vi "ma_FRF Function no State.vi"(0 "time signal X":waveform(dbl), 1 "time signal Y":waveform(dbl), 2 "window parameter":dbl=nan, 3 "window":T3=1 items=["Rectangle"=0, "Hanning"=1, "Hamming"=2, "Blackman-Harris"=3, "Exact Blackman"=4, "Blackman"=5, "Flat Top"=6, "4 Term B-Harris "=7, "7 Term B-Harris"=8, "Low Sidelobe"=9, "Blackman Nuttall"=11, "Triangle"=30, "Bartlett-Hanning"=31, "Bohman"=32, "Parzen"=33, "Welch"=34, "Kaiser"=60, "Dolph-Chebyshev"=61, "Gaussian"=62], 4 "view":T1, 5 "error in (no error)":errorcluster, 6 "restart averaging (F)":bool, 7 "averaging parameters":T5={"averaging mode"=enum."No averaging", "weighting mode"=enum."Exponential", "number of averages"=10} {"number of averages" min=1}, 8 "mag-phase":bool, 9 "state info":T2 {"Syy" format="%0.2f"; "Sxy" format="%0.2f"; "Sy" format="%0.2f"; "Sxx" format="%0.2f"; "avgs completed" format="%0.2f"; "df" format="%0.2f"; "Sx" format="%0.2f"; "spectrum parameters"."window" items=["Rectangle"=0, "Hanning"=1, "Hamming"=2, "Blackman-Harris"=3, "Exact Blackman"=4, "Blackman"=5, "Flat Top"=6, "4 Term B-Harris "=7, "7 Term B-Harris"=8, "Low Sidelobe"=9, "Blackman Nuttall"=11, "Triangle"=30, "Bartlett-Hanning"=31, "Bohman"=32, "Parzen"=33, "Welch"=34, "Kaiser"=60, "Dolph-Chebyshev"=61, "Gaussian"=62]; "dt" format="%0.2f"; "timestamp" format="%0.2f"; "dt history" format="%0.2f"; "t0 history" format="%0.2f"}, 11 "FRF Mode":enum16{"H1", "H2", "H3"}(ring)) -> (12 "averaging done":bool, 13 "state info out":T2 {"Syy" format="%0.2f"; "Sxy" format="%0.2f"; "Sy" format="%0.2f"; "Sxx" format="%0.2f"; "avgs completed" format="%0.2f"; "df" format="%0.2f"; "Sx" format="%0.2f"; "spectrum parameters"."window" items=["Rectangle"=0, "Hanning"=1, "Hamming"=2, "Blackman-Harris"=3, "Exact Blackman"=4, "Blackman"=5, "Flat Top"=6, "4 Term B-Harris "=7, "7 Term B-Harris"=8, "Low Sidelobe"=9, "Blackman Nuttall"=11, "Triangle"=30, "Bartlett-Hanning"=31, "Bohman"=32, "Parzen"=33, "Welch"=34, "Kaiser"=60, "Dolph-Chebyshev"=61, "Gaussian"=62]; "dt" format="%0.2f"; "timestamp" format="%0.2f"; "dt history" format="%0.2f"; "t0 history" format="%0.2f"}, 14 "real or mag":cluster{"f0":dbl, "df":dbl, "real or mag":dbl[]} {"real or mag" format="%.2p"; "f0" format="%0.2p"; "df" format="%0.2p"}, 15 "imag or phase":T4 {"imag or phase" format="%.2p"; "f0" format="%0.2p"; "df" format="%0.2p"}, 17 "coherence":cluster{"f0":dbl, "df":dbl, "coherence":dbl[]}, 18 "averages completed":dbl format="%.2p", 19 "error out":errorcluster)   [LabVIEW 2020, in "NI_MAPro.lvlib"]
doc: "Computes the frequency response and the coherence based on the input signals. Results are returned as <B>real part</B>, <B>imaginary part</B>, and <B>coherence</B>."
uses:
  NI_MAPro.lvlib
  windowTd.ctl
  2-chan State.ctl
  NI_AALPro.lvlib
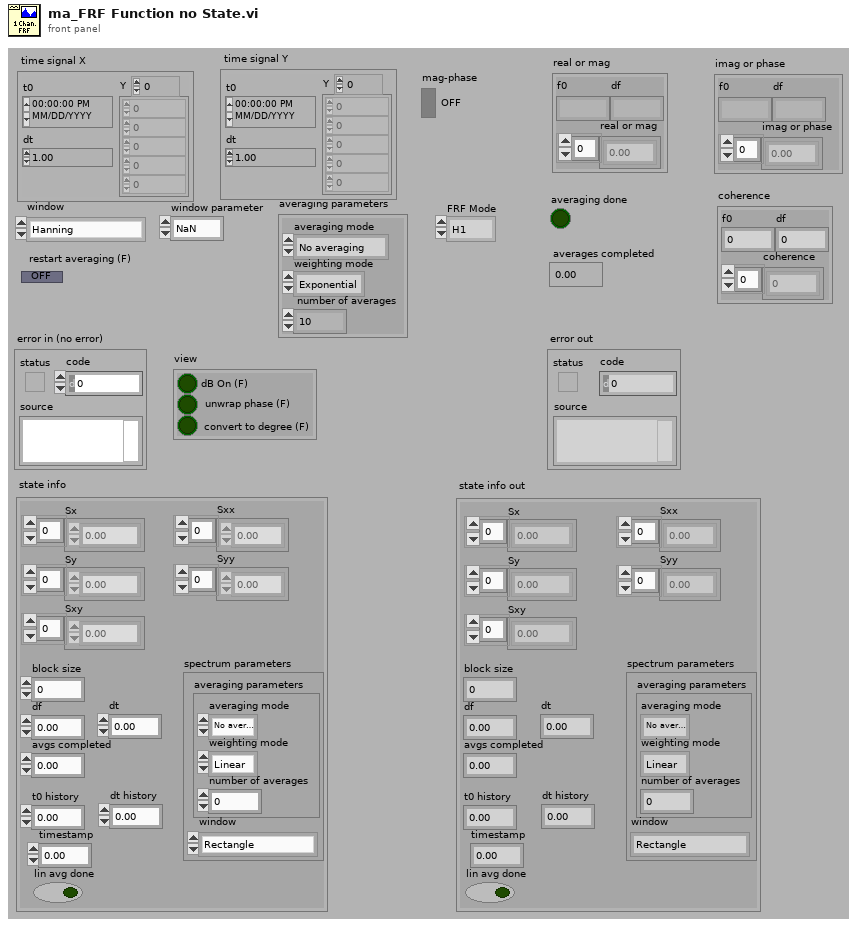
[diagram p1: front panel]
types:
  T1 = cluster{"dB On (F)":bool, "unwrap phase (F)":bool, "convert to degree (F)":bool}
  T2 = typedef "NI_MAPro.lvlib/2-chan State.ctl" = cluster{"Sx":cdb[], "Sy":cdb[], "Sxx":dbl[], "Syy":dbl[], "Sxy":cdb[], "block size":i32, "df":dbl, "dt":dbl, "avgs completed":dbl, "spectrum parameters":cluster{"averaging parameters":cluster{"averaging mode":enum16{"No averaging", "Vector averaging", "RMS averaging", "Peak hold"}, "weighting mode":enum16{"Linear", "Exponential"}, "number of averages":u32}, "window":T3}, "lin avg done":bool, "t0 history":dbl, "dt history":dbl, "timestamp":dbl}
  T3 = typedef "NI_AALPro.lvlib/windowTd.ctl" = u32
  T4 = cluster{"f0":dbl, "df":dbl, "imag or phase":dbl[]}
  T5 = cluster{"averaging mode":enum16{"No averaging", "Vector averaging", "RMS averaging", "Peak hold"}, "weighting mode":enum16{"Linear", "Exponential"}, "number of averages":u32}
  T6 = enum16{"FFT spectrum", "Power spectrum", "Cross spectrum", "Frequency response"}
  T7 = enum16{"No averaging", "Vector averaging", "RMS averaging", "Peak hold"}
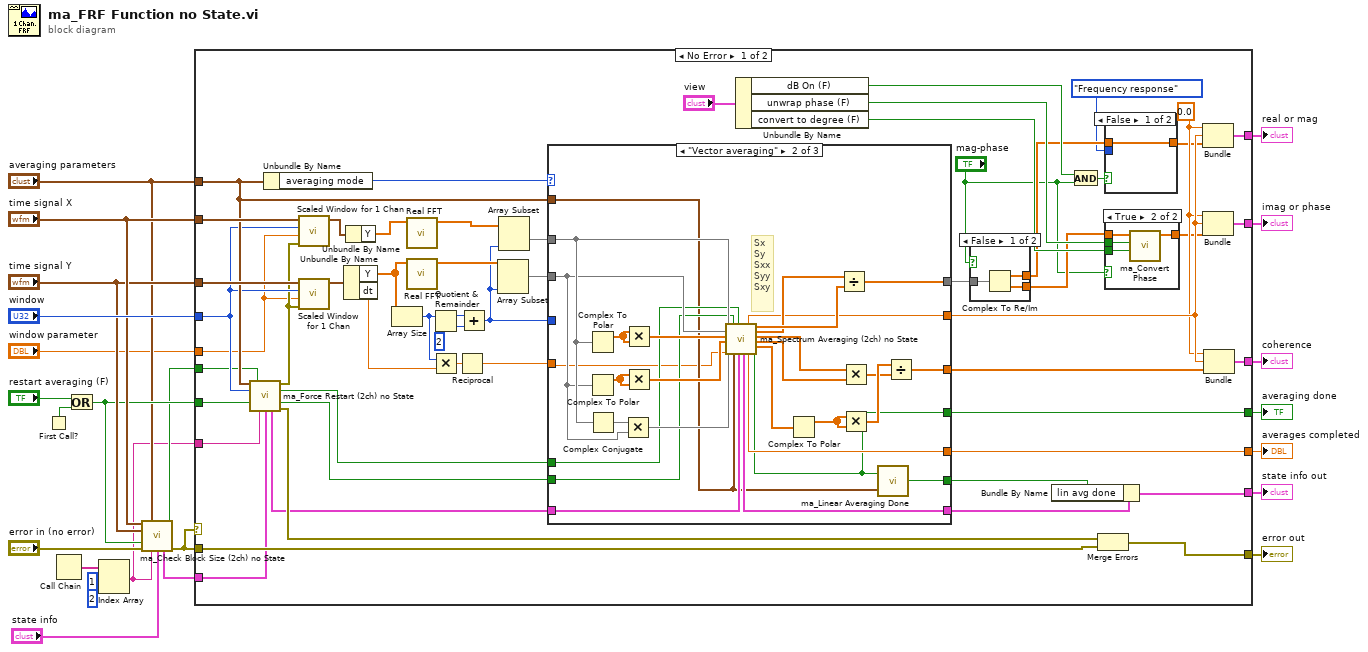
[diagram p0: block diagram]
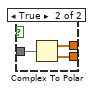
[diagram p2: hidden frame]
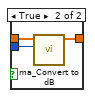
[diagram p4: hidden frame]
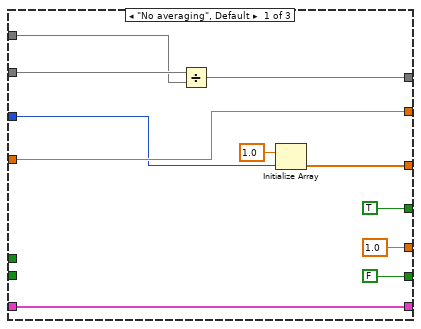
[diagram p5: hidden frame]
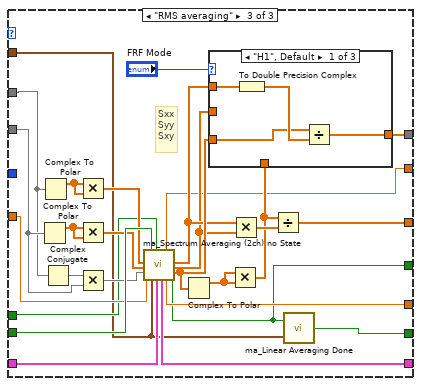
[diagram p6: hidden frame]
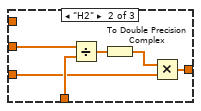
[diagram p7: hidden frame]
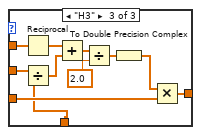
[diagram p8: hidden frame]
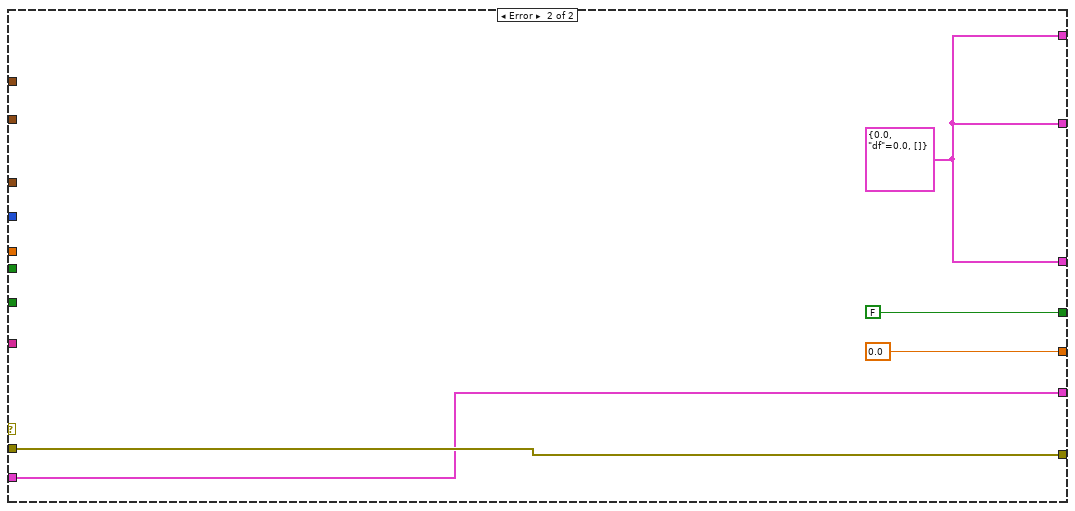
[diagram p9: hidden frame]
diagram:
  n1 = First Call?() -> (First Call?: T/F=w21:bool)
  n2 = Call Chain() -> (call chain=w6:string[])
  n3 = Or(x="restart averaging (F)", y=w21) -> (x .or. y?=w17:bool)
  n4 = Index Array(array=w6, index #1=1 ("Index"), index #2=2 ("Index")) -> (element #1=w5:string)  [unwired: 1 out]
  n5 = call "ma_Check Block Size (2ch) no State.vi"("time signal X"="time signal X", "averaging parameters"="averaging parameters", "time signal Y"="time signal Y", "restart averaging (F)"=w17, "error in"="error in (no error)", "caller VI name"=w5, "state info"="state info") -> ("force restart averaging"=w9:bool, "state info out"=w3:T2, "error out"=w14:errorcluster)  [unwired: 6 out]
  n6 = case shown="No Error" w14 {
    tunnel: [w80 0.0 ("averages completed")] -> w24
    tunnel: "time signal X" -> [w79 _]
    tunnel: "time signal Y" -> [w78 _]
    tunnel: [w77 FALSE ("averaging done")] -> w23
    tunnel: "averaging parameters" -> [w76 _]
    tunnel: "window" -> [w75 _]
    tunnel: w17 -> [w74 _]
    tunnel: [w67 w187] -> w15
    tunnel: w14 -> [w65 w187]
    tunnel: [w73 w185] -> w12
    tunnel: [w72 w185] -> w11
    tunnel: [w68 w185] -> w10
    tunnel: w5 -> [w64 _]
    tunnel: w9 -> [w63 _]
    tunnel: w3 -> [w62 w183]
    tunnel: [w39 w183] -> w2
    tunnel: "window parameter" -> [w25 _]
    frame No Error {
      w69 = 0.0
      n7 = call "ma_Force Restart (2ch) no State.vi"("averaging parameters"=w76, "force restart averaging in"=w63, "window"=w75, "restart averaging (F)"=w74, "caller VI name"=w64, "state info"=w62) -> ("skip processing"=w59:errorcluster, "force restart averaging"=w57:bool, "retrieve last spectrum"=w56:bool, "state info out"=w41:T2, "error out"=w66:errorcluster)  [unwired: 1 in, 4 out]
      n8 = Unbundle By Name(w76) -> ("averaging mode"=w58:T7)
      n9 = call "Scaled Window for 1 Chan.vi"("error in (no error)"=w59, "window parameter"=w25, "window"=w75, "signal in"=w79) -> ("signal out"=w60:waveform(dbl))  [unwired: 5 in, 2 out]
      n10 = call "Scaled Window for 1 Chan.vi"("error in (no error)"=w59, "window parameter"=w25, "window"=w75, "signal in"=w78) -> ("signal out"=w61:waveform(dbl))  [unwired: 5 in, 2 out]
      n11 = Unbundle By Name(w61) -> ("Y"=w46:dbl[], "dt"=w47:dbl)
      n12 = Unbundle By Name(w60) -> ("Y"=w45:dbl[])
      n13 = Array Size(array=w46) -> (size(s)=w55:i32)
      n14 = call "Real FFT.vi"("X"=w45) -> ("FFT {X}"=w53:cdb[])  [unwired: 9 in, 1 out]
      n15 = call "Real FFT.vi"("X"=w46) -> ("FFT {X}"=w54:cdb[])  [unwired: 9 in, 1 out]
      n16 = Quotient & Remainder(x=w55, y=2) -> (x-y*floor(x/y)=w50:i32, floor(x/y)=w49:i32)
      n17 = Multiply(x=w55, y=w47) -> (x*y=w52:dbl)
      n18 = Reciprocal(x=w52) -> (1/x=w48:dbl)
      n19 = Add(x=w50, y=w49) -> (x+y=w42:i32)
      n20 = Array Subset(array=w54, length=w42) -> (w43:cdb[])  [unwired: 1 in]
      n21 = Array Subset(array=w53, length=w42) -> (w44:cdb[])  [unwired: 1 in]
      n22 = case shown="\"Vector averaging\"" w58 {
        tunnel: [w100 w114 w137] -> w70
        tunnel: w57 -> [_ w115 w142]
        tunnel: w76 -> [_ w108 w135]
        tunnel: [1.0 ("averages completed") w116 w147] -> w80
        tunnel: [w105 w129 w160] -> w71
        tunnel: [TRUE ("averaging done") w113 w138] -> w77
        tunnel: w56 -> [_ w109 w148]
        tunnel: [FALSE ("linear averaging done") w131 w159] -> w40
        tunnel: w44 -> [w99 w126 w154]
        tunnel: w43 -> [w101 w125 w155]
        tunnel: w48 -> [w100 w107 w143]
        tunnel: w42 -> [w98 _ _]
        tunnel: w41 -> [w97 w112 w150]
        tunnel: [w97 w111 w149] -> w38
        tunnel: [w96 w110 w136] -> w30
        frame "No averaging", Default {
          n23 = Divide(x=w101, y=w99) -> (x/y=w96:cdb[])
          n24 = Initialize Array(1.0, w98) -> (w105:dbl[])
        }
        frame "Vector averaging" {
          # "Sx\nSy\nSxx\nSyy\nSxy"
          n25 = Complex To Polar(r * e^(i*theta)=w126) -> (r=w128:dbl[])  [unwired: 1 out]
          n26 = Complex To Polar(r * e^(i*theta)=w125) -> (r=w127:dbl[])  [unwired: 1 out]
          n27 = Complex Conjugate(1:w126) -> (0:w130:cdb[])
          n28 = Multiply(x=w130, y=w125) -> (x*y=w122:cdb[])
          n29 = Multiply(x=w128, y=w128) -> (x*y=w124:dbl[])
          n30 = Multiply(x=w127, y=w127) -> (x*y=w123:dbl[])
          n31 = call "ma_Spectrum Averaging (2ch) no State.vi"("Sx"=w126, "Sy"=w125, "Sxx"=w124, "Syy"=w123, "Sxy"=w122, "df"=w107, "retrieve last spectrum (F)"=w109, "averaging parameters"=w108, "restart averaging (F)"=w115, "state info"=w112) -> ("state info out"=w111:T2, "df"=w114:dbl, "averages completed"=w116:dbl, "avg Sx"=w121:cdb[], "avg Sy"=w120:cdb[], "avg Sxx"=w119:dbl[], "avg Syy"=w118:dbl[], "avg Sxy"=w117:cdb[], "averaging done"=w113:bool)  [unwired: 1 in]
          n32 = Complex To Polar(r * e^(i*theta)=w117) -> (r=w132:dbl[])  [unwired: 1 out]
          n33 = Divide(x=w120, y=w121) -> (x/y=w110:cdb[])
          n34 = Multiply(x=w119, y=w118) -> (x*y=w133:dbl[])
          n35 = Multiply(x=w132, y=w132) -> (x*y=w134:dbl[])
          n36 = call "ma_Linear Averaging Done.vi"("averaging parameters"=w108, "averaging done"=w113) -> ("linear averaging done"=w131:bool)
          n37 = Divide(x=w134, y=w133) -> (x/y=w129:dbl[])
        }
        frame "RMS averaging" {
          # "Sxx\nSyy\nSxy"
          n38 = Complex To Polar(r * e^(i*theta)=w155) -> (r=w156:dbl[])  [unwired: 1 out]
          n39 = Complex To Polar(r * e^(i*theta)=w154) -> (r=w157:dbl[])  [unwired: 1 out]
          n40 = Complex Conjugate(1:w154) -> (0:w158:cdb[])
          n41 = Multiply(x=w157, y=w157) -> (x*y=w146:dbl[])
          n42 = Multiply(x=w156, y=w156) -> (x*y=w145:dbl[])
          n43 = Multiply(x=w158, y=w155) -> (x*y=w144:cdb[])
          n44 = call "ma_Spectrum Averaging (2ch) no State.vi"("Sxx"=w146, "Syy"=w145, "Sxy"=w144, "df"=w143, "retrieve last spectrum (F)"=w148, "averaging parameters"=w135, "restart averaging (F)"=w142, "state info"=w150) -> ("state info out"=w149:T2, "df"=w137:dbl, "averages completed"=w147:dbl, "avg Sxx"=w140:dbl[], "avg Syy"=w139:dbl[], "avg Sxy"=w141:cdb[], "averaging done"=w138:bool)  [unwired: 3 in, 2 out]
          n45 = Complex To Polar(r * e^(i*theta)=w141) -> (r=w152:dbl[])  [unwired: 1 out]
          n46 = Multiply(x=w152, y=w152) -> (x*y=w153:dbl[])
          n47 = case shown="\"H1\", Default" "FRF Mode" {
            tunnel: w140 -> [w165 _ w174]
            tunnel: [w164 w170 w175] -> w136
            tunnel: w139 -> [_ w169 w173]
            tunnel: w141 -> [w162 w166 w176]
            tunnel: w153 -> [_ w168 w172]
            frame "H1", Default {
              n48 = To Double Precision Complex(1:w165) -> (0:w163:cdb[])
              n49 = Divide(x=w162, y=w163) -> (x/y=w164:cdb[])
            }
            frame "H2" {
              n50 = Divide(x=w169, y=w168) -> (x/y=w171:dbl[])
              n51 = To Double Precision Complex(1:w171) -> (0:w167:cdb[])
              n52 = Multiply(x=w167, y=w166) -> (x*y=w170:cdb[])
            }
            frame "H3" {
              n53 = Reciprocal(x=w174) -> (1/x=w177:dbl[])
              n54 = Divide(x=w173, y=w172) -> (x/y=w178:dbl[])
              n55 = Add(x=w177, y=w178) -> (x+y=w179:dbl[])
              n56 = Divide(x=w179, y=2.0) -> (x/y=w181:dbl[])
              n57 = To Double Precision Complex(1:w181) -> (0:w182:cdb[])
              n58 = Multiply(x=w182, y=w176) -> (x*y=w175:cdb[])
            }
          }
          n59 = Multiply(x=w140, y=w139) -> (x*y=w161:dbl[])
          n60 = Divide(x=w153, y=w161) -> (x/y=w160:dbl[])
          n61 = call "ma_Linear Averaging Done.vi"("averaging parameters"=w135, "averaging done"=w138) -> ("linear averaging done"=w159:bool)
        }
      }
      n62 = Unbundle By Name("view") -> ("dB On (F)"=w34:bool, "unwrap phase (F)"=w33:bool, "convert to degree (F)"=w32:bool)
      n63 = case shown="False" "mag-phase" {
        tunnel: w30 -> [w83 w86]
        tunnel: [w82 w85] -> w29
        tunnel: [w81 w84] -> w28
        frame False {
          n64 = Complex To Re/Im(x + iy=w83) -> (x=w82:dbl[], y=w81:dbl[])
        }
        frame True {
          n65 = Complex To Polar(r * e^(i*theta)=w86) -> (r=w85:dbl[], theta=w84:dbl[])
        }
      }
      n66 = Bundle By Name(cluster=w38, "lin avg done"=w40) -> (w39:T2)
      n67 = And(x=w34, y="mag-phase") -> (x .and. y?=w35:bool)
      n68 = Merge Errors(w66, w65) -> (w67:errorcluster)
      n69 = case shown="False" w35 {
        tunnel: [w92 w94] -> w36
        tunnel: w29 -> [w92 w95]
        tunnel: T6."Frequency response" ("spectrum type") -> [_ w93]
        frame False {
        }
        frame True {
          n70 = call "ma_Convert to dB.vi"("spectrum type"=w93, "spectrum"=w95) -> ("spectrum in dB"=w94:dbl[])  [unwired: 9 out]
        }
      }
      n71 = case shown="True" "mag-phase" {
        tunnel: [w87 w88] -> w31
        tunnel: w28 -> [w87 w91]
        tunnel: w33 -> [_ w90]
        tunnel: w32 -> [_ w89]
        frame False {
        }
        frame True {
          n72 = call "ma_Convert Phase.vi"("convert to degree (F)"=w89, "unwrap phase (F)"=w90, "phase (radian)"=w91) -> ("scaled phase"=w88:dbl[])  [unwired: 3 in, 5 out]
        }
      }
      n73 = Bundle(w69, "df"=w70, "spectrum in dB"=w36) -> (w73:cluster{dbl, "df":dbl, "spectrum in dB":dbl[]})  [unwired: 1 out]
      n74 = Bundle(w69, "df"=w70, "scaled phase"=w31) -> (w72:cluster{dbl, "df":dbl, "scaled phase":dbl[]})  [unwired: 1 out]
      n75 = Bundle(w69, "df"=w70, w71) -> (w68:cluster{dbl, "df":dbl, dbl[]})  [unwired: 1 out]
    }
    frame Error {
      w185 = cluster{dbl, "df":dbl, dbl[]} {0.0, "df"=0.0, []}
    }
  }
  "averages completed" <- w24
  "error out" <- w15
  "averaging done" <- w23
  "coherence" <- w10
  "imag or phase" <- w11
  "real or mag" <- w12
  "state info out" <- w2
